vi "App Stop.vi"(8 "error in (no error)":errorcluster, 11 "VolatusCoreTask in":refnum<class "VolatusCoreTask.lvclass">) -> (0 "error out":errorcluster, 3 "VolatusCoreTask out":refnum<class "VolatusCoreTask.lvclass">)   [LabVIEW 2020, in "Volatus.lvlib" / "VolatusCoreTask.lvclass"]
uses:
  VolatusCoreTask.lvclass
  VolatusCoreTask.lvclass/VolatusCoreTask.ctl
  App/App.lvclass
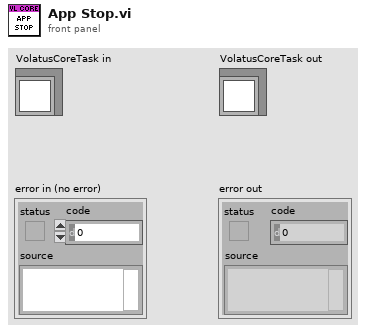
[diagram p1: front panel]
types:
  T1 = typedef "Volatus.lvlib/Core APIs.ctl" = cluster{"VolatusAPI":refnum<class "VolatusAPI.lvclass">, "EventAPI":refnum<class "EventAPI.lvclass">}
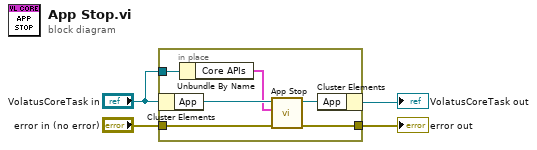
[diagram p0: block diagram]
diagram:
  n1 = in-place {
    in-place-border: "error in (no error)" -> [w10]
    in-place-border: [w9] -> w3
    in-place-border: "VolatusCoreTask in" -> [w7]
    n2 = in-place-cluster #1("VolatusCoreTask in") -> ("App"=w8:refnum<class "App.lvclass">)
    n3 = Unbundle By Name(w7) -> ("Core APIs"=w6:T1)
    n4 = call-dynamic "App Stop.vi"("error in (no error)"=w10, "Core APIs"=w6, "App in"=w8) -> ("error out"=w9:errorcluster, "App out"=w5:refnum<class "App.lvclass">)  [unwired: 7 in]
    n5 = in-place-cluster #1("App"=w5) -> (→"VolatusCoreTask out":refnum<class "VolatusCoreTask.lvclass">)
  }
  "error out" <- w3
